vi "Actor Receive.vi"(11 "Self Actor in":refnum<class "Self Actor.lvclass">) -> (0 "error out":errorcluster, 2 "Msg":refnum<class "Msg Strategy.lvclass">)   [LabVIEW 2021, in "LVCAM.lvlib" / "Self Actor.lvclass"]
uses:
  Self Actor.lvclass
  Msg Strategy/Msg Strategy.lvclass
  Self Actor.lvclass/Self Actor.ctl
  Self Actor State/Self Actor State.lvclass
  LVCAM.lvlib
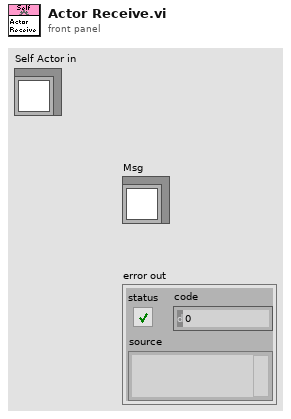
[diagram p1: front panel]
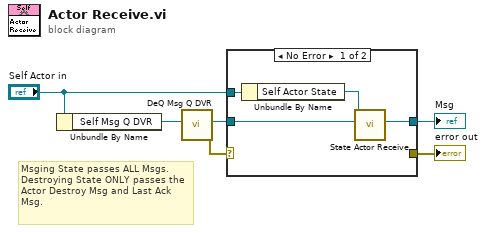
[diagram p0: block diagram]
diagram:
  # "Msging State passes ALL Msgs.\nDestroying State ONLY passes the Actor Destroy Msg and Last Ack Msg."
  n1 = Unbundle By Name("Self Actor in") -> ("Self Msg Q DVR"=w5:refnum<data-value>)
  n2 = call "DeQ Msg Q DVR.vi"("Msg Q DVR"=w5) -> ("error out"=w4:errorcluster, "Msg"=w2:refnum<class "Msg Strategy.lvclass">)  [unwired: 9 in]
  n3 = case shown="No Error" w4 {
    selector: w4 -> [_ w11]
    tunnel: [_ w11] -> w6
    tunnel: [w7 _] -> w3
    tunnel: w2 -> [w8 _]
    tunnel: "Self Actor in" -> [w10 _]
    frame No Error {
      n4 = Unbundle By Name(w10) -> ("Self Actor State"=w9:refnum<class "Self Actor State.lvclass">)
      n5 = call-dynamic "State Actor Receive.vi"("Msg in"=w8, "Self Actor State in"=w9) -> ("Msg out"=w7:refnum<class "Msg Strategy.lvclass">)  [unwired: 9 in]
    }
    frame Error {
    }
  }
  "Msg" <- w3
  "error out" <- w6
